vi "Uplink MICS.vi"(8 "Error In":errorcluster, 10 "MICS Block Size":u8, 11 "Reference In":i32) -> (0 "Error Out":errorcluster, 2 "Uplink":u8[][](array[numeric]) format="%02x", 3 "Reference Out":i32)   [LabVIEW 2009]
uses:
  Reference.vi
panel:
  # "UPLINK"
  # "Block 1"
  # "Block 2"
  # "Block 3"
  # "Block 4"
  # "b1"
  # "b2"
  # "b3"
  # "b4"
  # "b5"
  # "b6"
  # "b7"
  # "b8"
  # "b9"
  # "b10"
  # "b11"
  # "b12"
  # "b13"
  # "b14"
  # "b15"
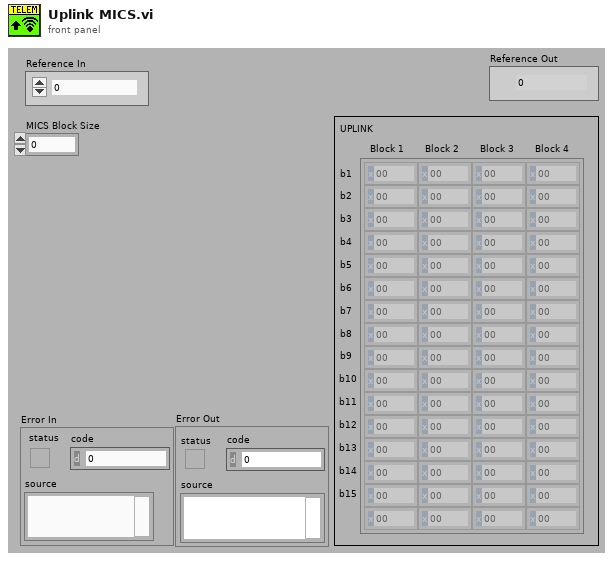
[diagram p1: front panel]
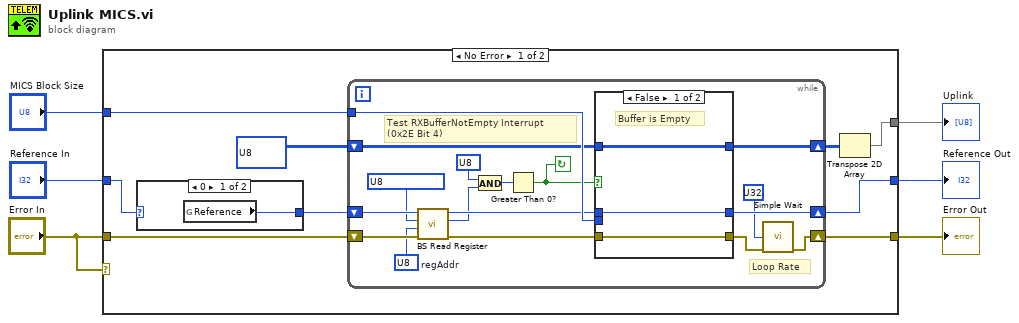
[diagram p0: block diagram]
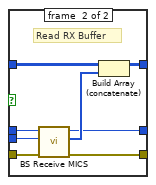
[diagram p3: hidden frame]
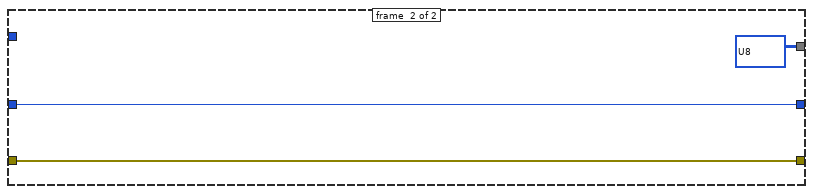
[diagram p4: hidden frame]
diagram:
  n1 = case shown="No Error" "Error In" {
    tunnel: "Error In" -> [w10 w48]
    tunnel: "Reference In" -> [w8 w46]
    tunnel: [w15 w48] -> w5
    tunnel: [w12 u8[][] ? ("buf")] -> w4
    tunnel: [w14 w46] -> w2
    tunnel: "MICS Block Size" -> [w7 _]
    frame #0 {
      n2 = case shown="0" w8 {
        selector: w8 -> [_ w17]
        tunnel: [w16 w17] -> w9
        frame #0 {
          n3 = global read "Reference.vi" "Reference"() -> (w16:i32)
        }
        frame #1 {
        }
      }
      n4 = while {
        tunnel: w7 -> [w34]
        shift-right: [w31] -> w14
        shift-left: w9 -> [w30]
        shift-right: [w20] -> w15
        shift-left: w10 -> [w29]
        shift-right: [w33] -> w13
        shift-left: u8[][] ? -> [w32]
        stop <- w21 continue-if-true
        w25 = u8 ?  # regAddr
        w26 = u8 ? items=["Base Station", "Implant"] ("Board Type")
        # "Loop Rate"
        # "Test RXBufferNotEmpty Interrupt\n(0x2E Bit 4)"
        n5 = call <vilib>:"BS Read Register.vi"("Error In"=w29, "regAddr"=w25, "Board Type"=w26, "Reference In"=w30) -> ("Error Out"=w28:errorcluster, "regVal"=w24:u8, "Reference Out"=w27:i32)  [unwired: 4 in]
        n6 = And(x=u8 ? ("regAddr"), y=w24) -> (x .and. y?=w22:u8)
        n7 = Greater Than 0?(x=w22) -> (x > 0?=w21:bool)
        n8 = case shown="False" w21 {
          tunnel: w27 -> [w36 w45]
          tunnel: w28 -> [w35 w44]
          tunnel: w34 -> [_ w43]
          tunnel: [w37 w41] -> w33
          tunnel: w32 -> [w37 w40]
          tunnel: [w35 w39] -> w19
          tunnel: [w36 w38] -> w31
          frame #0 {
            # "Buffer is Empty"
          }
          frame #1 {
            # "Read RX Buffer"
            n9 = call <vilib>:"BS Receive MICS.vi"("Error In"=w44, "Packet Length"=w43, "Reference In"=w45) -> ("Error Out"=w39:errorcluster, "buf"=w42:u8[], "Reference Out"=w38:i32)  [unwired: 3 in, 1 out]
            n10 = Build Array (concatenate)(w40, w42) -> (w41:u8[][])
          }
        }
        n11 = call "Simple Wait.vi"("mS"=u32 ?, "error in"=w19) -> ("error out"=w20:errorcluster)  [unwired: 12 in, 1 out]
      }
      n12 = Transpose 2D Array(2D array=w13) -> (transposed array=w12:u8[][])
    }
    frame #1 {
    }
  }
  "Error Out" <- w5
  "Uplink" <- w4
  "Reference Out" <- w2
